vi "Get Robot Config.vi"() -> (12 "Idle Ramping Table":T1(array[cluster]), 13 "Cascade FeedForward Constants":cluster{"kA":dbl, "kS":dbl, "kG":dbl, "kV":dbl}, 14 "Manipulator Config":T2, 15 "Intake Presets":T5(array[cluster]), 16 "Scoring Overrides Ramping Table":T1(array[cluster]), 17 "Color":u32(colorbox)=8978432, 18 "Shoot Cube Config":T4, 19 "Score Ramping Table":T3(array[cluster]))   [LabVIEW 2020]
uses:
  <vilib>/Rock Robotics/Network Tables/NT Read Number.vi
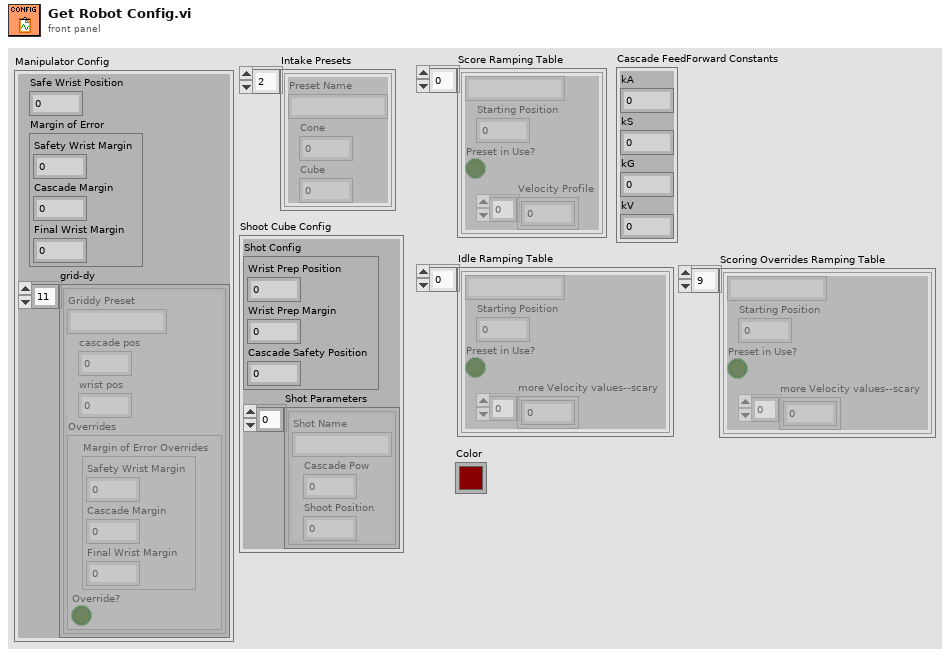
[diagram p1: front panel]
types:
  T1 = cluster{string, "Starting Position":dbl, "Preset in Use?":bool, "more Velocity values--scary":dbl[]}[]
  T2 = cluster{"Safe Wrist Position":dbl, "Margin of Error":cluster{"Safety Wrist Margin":dbl, "Cascade Margin":dbl, "Final Wrist Margin":dbl}, "grid-dy":cluster{"Griddy Preset":string, "cascade pos":dbl, "wrist pos":dbl, "Overrides":cluster{"Margin of Error Overrides":cluster{"Safety Wrist Margin":dbl, "Cascade Margin":dbl, "Final Wrist Margin":dbl}, "Override?":bool}}[]}
  T3 = cluster{string, "Starting Position":dbl, "Preset in Use?":bool, "Velocity Profile":dbl[]}[]
  T4 = cluster{"Shot Config":cluster{"Wrist Prep Position":dbl, "Wrist Prep Margin":dbl, "Cascade Safety Position":dbl}, "Shot Parameters":cluster{"Shot Name":string, "Cascade Pow":dbl, "Shoot Position":dbl}[]}
  T5 = cluster{"Preset Name":string, "Cone":dbl, "Cube":dbl}[]
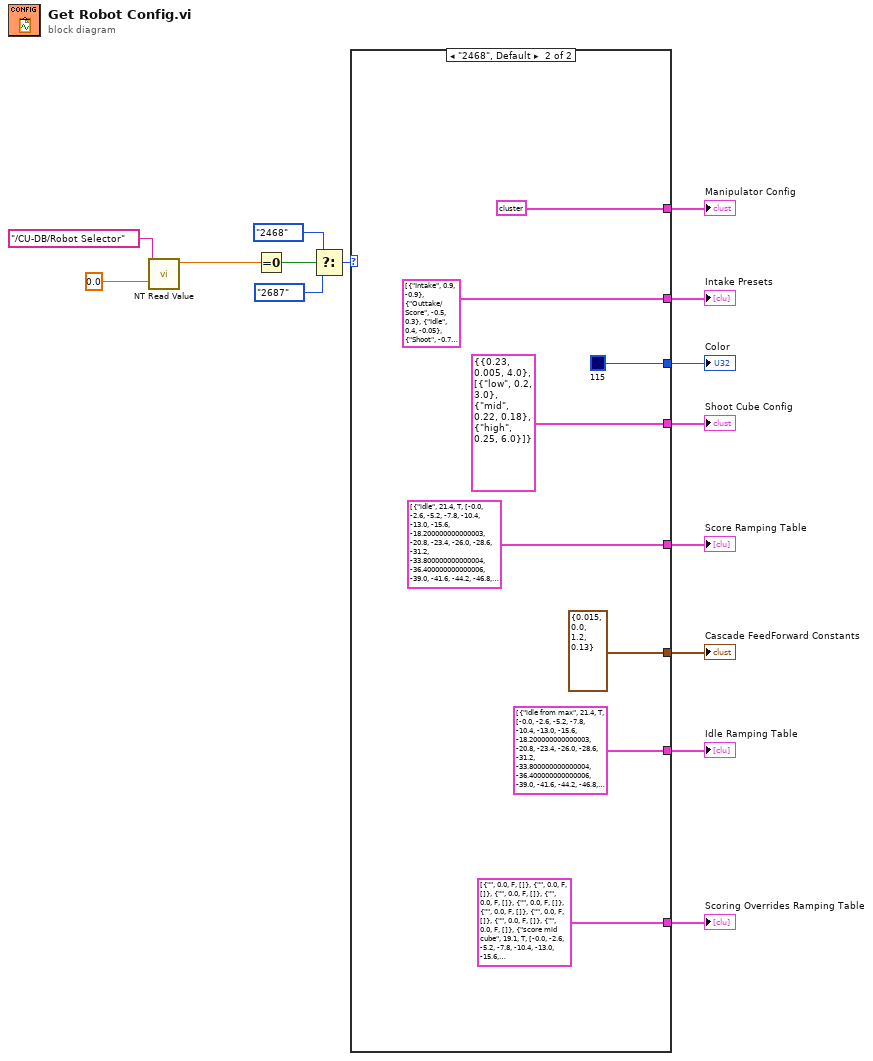
[diagram p0: block diagram]
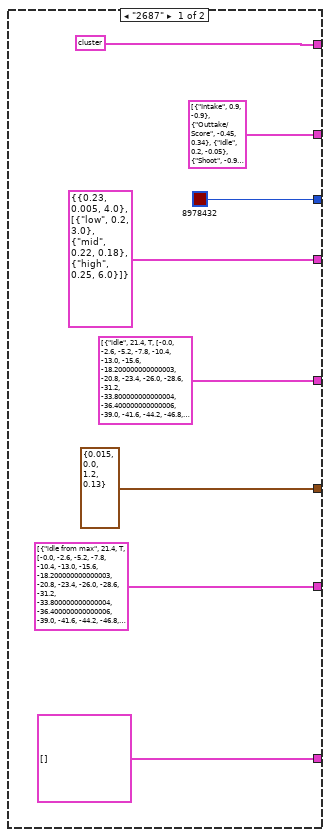
[diagram p2: hidden frame]
diagram:
  n1 = call-poly <vilib>:"NT Read Value.vi"("default value"=0.0, "name"="/CU-DB/Robot Selector") -> ("value"=w14:dbl)  [unwired: 7 in, 2 out]
  n2 = Equal To 0?(x=w14) -> (x = 0?=w13:bool)
  n3 = Select(t=enum16{"2468", "2687"}."2468", s=w13, f=enum16{"2468", "2687"}."2687") -> (s? t:f=w10:enum16{"2468", "2687"})
  n4 = case shown="\"2468\", Default" w10 {
    tunnel: [T2 {"Safe Wrist Position"=0.35, "Margin of Error"={"Safety Wrist Margin"=0.3, "Cascade Margin"=2.0, "Final Wrist Margin"=0.03}, "grid-dy"=[{"Griddy Preset"="idle", "cascade pos"=0.0, "wrist pos"=0.25, "Overrides"={"Margin of Error Overrides"={"Safety Wrist Margin"=0.3, "Cascade Margin"=2.0, "Final Wrist Margin"=0.03}, "Override?"=FALSE}}, {"Griddy Preset"="intake cone sideways", "cascade pos"=0.0, "wrist pos"=0.685, "Overrides"={"Margin of Error Overrides"={"Safety Wrist Margin"=0.3, "Cascade Margin"=2.0, "Final Wrist Margin"=0.03}, "Override?"=FALSE}}, {"Griddy Preset"="intake cone upright", "cascade pos"=6.5, "wrist pos"=0.75, "Overrides"={"Margin of Error Overrides"={"Safety Wrist Margin"=0.3, "Cascade Margin"=2.0, "Final Wrist Margin"=0.03}, "Override?"=FALSE}}, {"Griddy Preset"="intake cone feeder", "cascade pos"=0.0, "wrist pos"=0.42, "Overrides"={"Margin of Error Overrides"={"Safety Wrist Margin"=0.3, "Cascade Margin"=2.0, "Final Wrist Margin"=0.03}, "Override?"=FALSE}}, {"Griddy Preset"="intake cube feeder", "cascade pos"=0.0, "wrist pos"=0.2, "Overrides"={"Margin of Error Overrides"={"Safety Wrist Margin"=0.3, "Cascade Margin"=2.0, "Final Wrist Margin"=0.03}, "Override?"=FALSE}}, {"Griddy Preset"="intake cube", "cascade pos"=0.0, "wrist pos"=0.58, "Overrides"={"Margin of Error Overrides"={"Safety Wrist Margin"=0.3, "Cascade Margin"=2.0, "Final Wrist Margin"=0.03}, "Override?"=FALSE}}, {"Griddy Preset"="score low cone", "cascade pos"=0.0, "wrist pos"=0.5, "Overrides"={"Margin of Error Overrides"={"Safety Wrist Margin"=0.3, "Cascade Margin"=2.0, "Final Wrist Margin"=0.03}, "Override?"=FALSE}}, {"Griddy Preset"="score low cube", "cascade pos"=0.0, "wrist pos"=0.25, "Overrides"={"Margin of Error Overrides"={"Safety Wrist Margin"=0.3, "Cascade Margin"=2.0, "Final Wrist Margin"=0.03}, "Override?"=FALSE}}, {"Griddy Preset"="score mid cone", "cascade pos"=21.4, "wrist pos"=0.79, "Overrides"={"Margin of Error Overrides"={"Safety Wrist Margin"=0.3, "Cascade Margin"=13.0, "Final Wrist Margin"=0.03}, "Override?"=TRUE}}, {"Griddy Preset"="score mid cube", "cascade pos"=8.9, "wrist pos"=0.4, "Overrides"={"Margin of Error Overrides"={"Safety Wrist Margin"=0.3, "Cascade Margin"=2.0, "Final Wrist Margin"=0.03}, "Override?"=FALSE}}, {"Griddy Preset"="score high cone", "cascade pos"=21.4, "wrist pos"=0.62, "Overrides"={"Margin of Error Overrides"={"Safety Wrist Margin"=0.3, "Cascade Margin"=2.0, "Final Wrist Margin"=0.03}, "Override?"=FALSE}}, {"Griddy Preset"="score high cube", "cascade pos"=19.1, "wrist pos"=0.4, "Overrides"={"Margin of Error Overrides"={"Safety Wrist Margin"=0.3, "Cascade Margin"=2.0, "Final Wrist Margin"=0.03}, "Override?"=FALSE}}]} ("2468 Manipulator Config") T2 {"Safe Wrist Position"=0.35, "Margin of Error"={"Safety Wrist Margin"=0.3, "Cascade Margin"=2.0, "Final Wrist Margin"=0.03}, "grid-dy"=[{"Griddy Preset"="idle", "cascade pos"=0.0, "wrist pos"=0.25, "Overrides"={"Margin of Error Overrides"={"Safety Wrist Margin"=0.3, "Cascade Margin"=2.0, "Final Wrist Margin"=0.03}, "Override?"=FALSE}}, {"Griddy Preset"="intake cone sideways", "cascade pos"=0.0, "wrist pos"=0.69, "Overrides"={"Margin of Error Overrides"={"Safety Wrist Margin"=0.3, "Cascade Margin"=2.0, "Final Wrist Margin"=0.03}, "Override?"=FALSE}}, {"Griddy Preset"="intake cone upright", "cascade pos"=6.3, "wrist pos"=0.75, "Overrides"={"Margin of Error Overrides"={"Safety Wrist Margin"=0.3, "Cascade Margin"=2.0, "Final Wrist Margin"=0.03}, "Override?"=FALSE}}, {"Griddy Preset"="intake cone feeder", "cascade pos"=0.0, "wrist pos"=0.42, "Overrides"={"Margin of Error Overrides"={"Safety Wrist Margin"=0.3, "Cascade Margin"=2.0, "Final Wrist Margin"=0.03}, "Override?"=FALSE}}, {"Griddy Preset"="intake cube feeder", "cascade pos"=0.0, "wrist pos"=0.2, "Overrides"={"Margin of Error Overrides"={"Safety Wrist Margin"=0.3, "Cascade Margin"=2.0, "Final Wrist Margin"=0.03}, "Override?"=FALSE}}, {"Griddy Preset"="intake cube", "cascade pos"=0.0, "wrist pos"=0.59, "Overrides"={"Margin of Error Overrides"={"Safety Wrist Margin"=0.3, "Cascade Margin"=2.0, "Final Wrist Margin"=0.03}, "Override?"=FALSE}}, {"Griddy Preset"="score low cone", "cascade pos"=0.0, "wrist pos"=0.5, "Overrides"={"Margin of Error Overrides"={"Safety Wrist Margin"=0.3, "Cascade Margin"=2.0, "Final Wrist Margin"=0.03}, "Override?"=FALSE}}, {"Griddy Preset"="score low cube", "cascade pos"=0.0, "wrist pos"=0.25, "Overrides"={"Margin of Error Overrides"={"Safety Wrist Margin"=0.3, "Cascade Margin"=2.0, "Final Wrist Margin"=0.03}, "Override?"=FALSE}}, {"Griddy Preset"="score mid cone", "cascade pos"=21.4, "wrist pos"=0.82, "Overrides"={"Margin of Error Overrides"={"Safety Wrist Margin"=0.3, "Cascade Margin"=13.0, "Final Wrist Margin"=0.03}, "Override?"=TRUE}}, {"Griddy Preset"="score mid cube", "cascade pos"=8.9, "wrist pos"=0.38, "Overrides"={"Margin of Error Overrides"={"Safety Wrist Margin"=0.3, "Cascade Margin"=2.0, "Final Wrist Margin"=0.03}, "Override?"=FALSE}}, {"Griddy Preset"="score high cone", "cascade pos"=21.4, "wrist pos"=0.62, "Overrides"={"Margin of Error Overrides"={"Safety Wrist Margin"=0.3, "Cascade Margin"=2.0, "Final Wrist Margin"=0.03}, "Override?"=FALSE}}, {"Griddy Preset"="score high cube", "cascade pos"=19.1, "wrist pos"=0.4, "Overrides"={"Margin of Error Overrides"={"Safety Wrist Margin"=0.3, "Cascade Margin"=2.0, "Final Wrist Margin"=0.03}, "Override?"=FALSE}}]} ("2468 Manipulator Config")] -> w2
    tunnel: [T5 [{"Preset Name"="Intake", "Cone"=0.9, "Cube"=-0.9}, {"Preset Name"="Outtake/Score", "Cone"=-0.45, "Cube"=0.34}, {"Preset Name"="Idle", "Cone"=0.2, "Cube"=-0.05}, {"Preset Name"="Shoot", "Cone"=-0.9, "Cube"=0.9}] ("2687 Intake Presets") T5 [{"Preset Name"="Intake", "Cone"=0.9, "Cube"=-0.9}, {"Preset Name"="Outtake/Score", "Cone"=-0.5, "Cube"=0.3}, {"Preset Name"="Idle", "Cone"=0.4, "Cube"=-0.05}, {"Preset Name"="Shoot", "Cone"=-0.7, "Cube"=0.9}] ("2468 Intake Presets")] -> w9
    tunnel: [u32 8978432 ("Red") u32 115 ("Blue")] -> w8
    tunnel: [T4 {"Shot Config"={"Wrist Prep Position"=0.23, "Wrist Prep Margin"=0.005, "Cascade Safety Position"=4.0}, "Shot Parameters"=[{"Shot Name"="low", "Cascade Pow"=0.2, "Shoot Position"=3.0}, {"Shot Name"="mid", "Cascade Pow"=0.22, "Shoot Position"=0.18}, {"Shot Name"="high", "Cascade Pow"=0.25, "Shoot Position"=6.0}]} ("2687 Shoot Cube Config") T4 {"Shot Config"={"Wrist Prep Position"=0.23, "Wrist Prep Margin"=0.005, "Cascade Safety Position"=4.0}, "Shot Parameters"=[{"Shot Name"="low", "Cascade Pow"=0.2, "Shoot Position"=3.0}, {"Shot Name"="mid", "Cascade Pow"=0.22, "Shoot Position"=0.18}, {"Shot Name"="high", "Cascade Pow"=0.25, "Shoot Position"=6.0}]} ("2687 Shoot Cube Config")] -> w6
    tunnel: [T1 [{"idle", "Starting Position"=21.4, "Preset in Use?"=TRUE, "more Velocity values--scary"=[-0.0, -2.6, -5.2, -7.8, -10.4, -13.0, -15.6, -18.200000000000003, -20.8, -23.4, -26.0, -28.6, -31.2, -33.800000000000004, -36.400000000000006, -39.0, -41.6, -44.2, -46.8, -49.4, -52.0, -49.89880242347718, -47.29880242347717, -44.69880242347717, -42.098802423477174, -39.49880242347717, -36.89880242347717, -34.29880242347717, -31.698802423477165, -29.098802423477178, -26.498802423477176, -23.898802423477175, -21.29880242347717, -18.69880242347717, -16.098802423477167, -13.49880242347718, -10.898802423477179, -8.298802423477177, -5.698802423477169, -3.098802423477167, -0.49880242347716575]}, {"", "Starting Position"=0.0, "Preset in Use?"=FALSE, "more Velocity values--scary"=[]}, {"intake cone upright", "Starting Position"=0.0, "Preset in Use?"=TRUE, "more Velocity values--scary"=[0.0, 2.6, 5.2, 7.8, 10.4, 13.0, 15.6, 18.200000000000003, 20.8, 23.4, 26.0, 28.6, 28.26427345275879, 25.66427345275879, 23.064273452758783, 20.46427345275879, 17.864273452758788, 15.264273452758786, 12.664273452758792, 10.064273452758787, 7.4642734527587855, 4.864273452758791, 2.2642734527587898, -0.3357265472412152]}, {"", "Starting Position"=0.0, "Preset in Use?"=FALSE, "more Velocity values--scary"=[]}, {"", "Starting Position"=0.0, "Preset in Use?"=FALSE, "more Velocity values--scary"=[]}, {"", "Starting Position"=0.0, "Preset in Use?"=FALSE, "more Velocity values--scary"=[]}, {"", "Starting Position"=0.0, "Preset in Use?"=FALSE, "more Velocity values--scary"=[]}, {"", "Starting Position"=0.0, "Preset in Use?"=FALSE, "more Velocity values--scary"=[]}, {"score mid cone", "Starting Position"=0.0, "Preset in Use?"=TRUE, "more Velocity values--scary"=[0.0, 2.6, 5.2, 7.8, 10.4, 13.0, 15.6, 18.200000000000003, 20.8, 23.4, 26.0, 28.6, 31.2, 33.800000000000004, 36.400000000000006, 39.0, 41.6, 44.2, 46.8, 49.4, 49.98038995265961, 47.38038995265961, 44.780389952659604, 42.1803899526596, 39.58038995265961, 36.98038995265961, 34.380389952659606, 31.780389952659604, 29.1803899526596, 26.580389952659612, 23.98038995265961, 21.38038995265961, 18.780389952659604, 16.180389952659603, 13.580389952659601, 10.980389952659614, 8.380389952659613, 5.780389952659611, 3.1803899526596027, 0.5803899526596012]}, {"score mid cube", "Starting Position"=0.0, "Preset in Use?"=TRUE, "more Velocity values--scary"=[0.0, 2.6, 5.2, 7.8, 10.4, 13.0, 15.6, 18.200000000000003, 20.8, 23.4, 26.0, 28.6, 31.2, 32.683082771301265, 30.083082771301267, 27.48308277130127, 24.883082771301268, 22.283082771301267, 19.683082771301272, 17.083082771301267, 14.483082771301266, 11.883082771301272, 9.28308277130127, 6.683082771301265, 4.083082771301271, 1.4830827713012695, -1.116917228698732]}, {"score high cone", "Starting Position"=0.0, "Preset in Use?"=TRUE, "more Velocity values--scary"=[0.0, 1.6, 3.2, 4.8, 6.4, 8.0, 9.6, 11.200000000000001, 12.8, 14.399999999999999, 16.0, 17.6, 19.2, 20.8, 22.400000000000002, 24.0, 25.6, 27.200000000000003, 28.799999999999997, 30.4, 32.0, 33.6, 35.2, 36.800000000000004, 38.4, 40.0, 41.15264739990234, 39.55264739990234, 37.95264739990234, 36.352647399902345, 34.752647399902344, 33.15264739990234, 31.55264739990234, 29.95264739990234, 28.352647399902338, 26.752647399902347, 25.152647399902346, 23.552647399902344, 21.952647399902343, 20.35264739990234, 18.75264739990234, 17.15264739990235, 15.552647399902348, 13.952647399902347, 12.352647399902345, 10.752647399902344, 9.152647399902342, 7.552647399902348, 5.952647399902347, 4.352647399902345, 2.7526473999023438, 1.1526473999023423, -0.4473526000976591]}, {"score high cube", "Starting Position"=0.0, "Preset in Use?"=TRUE, "more Velocity values--scary"=[0.0, 2.6, 5.2, 7.8, 10.4, 13.0, 15.6, 18.200000000000003, 20.8, 23.4, 26.0, 28.6, 31.2, 33.800000000000004, 36.400000000000006, 39.0, 41.6, 44.2, 46.8, 49.4, 47.39819097518921, 44.798190975189215, 42.198190975189206, 39.598190975189205, 36.99819097518921, 34.39819097518921, 31.798190975189208, 29.198190975189206, 26.5981909751892, 23.998190975189214, 21.398190975189213, 18.79819097518921, 16.198190975189206, 13.598190975189205, 10.998190975189203, 8.398190975189216, 5.798190975189215, 3.1981909751892132, 0.5981909751892047]}] ("2687 Score Ramping Table") T1 [{"idle", "Starting Position"=21.4, "Preset in Use?"=TRUE, "more Velocity values--scary"=[-0.0, -2.6, -5.2, -7.8, -10.4, -13.0, -15.6, -18.200000000000003, -20.8, -23.4, -26.0, -28.6, -31.2, -33.800000000000004, -36.400000000000006, -39.0, -41.6, -44.2, -46.8, -49.4, -52.0, -49.89880242347718, -47.29880242347717, -44.69880242347717, -42.098802423477174, -39.49880242347717, -36.89880242347717, -34.29880242347717, -31.698802423477165, -29.098802423477178, -26.498802423477176, -23.898802423477175, -21.29880242347717, -18.69880242347717, -16.098802423477167, -13.49880242347718, -10.898802423477179, -8.298802423477177, -5.698802423477169, -3.098802423477167, -0.49880242347716575]}, {"", "Starting Position"=0.0, "Preset in Use?"=FALSE, "more Velocity values--scary"=[]}, {"intake cone upright", "Starting Position"=0.0, "Preset in Use?"=TRUE, "more Velocity values--scary"=[0.0, 1.26, 2.52, 3.78, 5.04, 6.300000000000001, 7.56, 8.82, 10.08, 11.34, 12.600000000000001, 13.86, 15.12, 16.38, 17.64, 18.9, 19.68469825029373, 18.42469825029373, 17.164698250293732, 15.90469825029373, 14.64469825029373, 13.384698250293733, 12.124698250293733, 10.864698250293731, 9.604698250293733, 8.344698250293732, 7.08469825029373, 5.824698250293729, 4.564698250293729, 3.3046982502937325, 2.0446982502937345, 0.784698250293733, -0.4753017497062686]}, {"", "Starting Position"=0.0, "Preset in Use?"=FALSE, "more Velocity values--scary"=[]}, {"", "Starting Position"=0.0, "Preset in Use?"=FALSE, "more Velocity values--scary"=[]}, {"", "Starting Position"=0.0, "Preset in Use?"=FALSE, "more Velocity values--scary"=[]}, {"", "Starting Position"=0.0, "Preset in Use?"=FALSE, "more Velocity values--scary"=[]}, {"", "Starting Position"=0.0, "Preset in Use?"=FALSE, "more Velocity values--scary"=[]}, {"score mid cone", "Starting Position"=0.0, "Preset in Use?"=TRUE, "more Velocity values--scary"=[0.0, 1.26, 2.52, 3.78, 5.04, 6.300000000000001, 7.56, 8.82, 10.08, 11.34, 12.600000000000001, 13.86, 15.12, 16.38, 17.64, 18.9, 20.16, 21.42, 22.68, 23.94, 25.200000000000003, 26.459999999999997, 27.72, 28.98, 30.24, 31.5, 32.76, 34.02, 35.28, 36.54, 35.63568778038025, 34.37568778038025, 33.11568778038025, 31.855687780380247, 30.595687780380246, 29.33568778038025, 28.07568778038025, 26.81568778038025, 25.555687780380246, 24.29568778038025, 23.035687780380247, 21.775687780380252, 20.51568778038025, 19.25568778038025, 17.995687780380248, 16.735687780380246, 15.475687780380248, 14.215687780380254, 12.955687780380252, 11.69568778038025, 10.435687780380249, 9.175687780380247, 7.915687780380246, 6.655687780380244, 5.395687780380243, 4.135687780380245, 2.8756877803802396, 1.6156877803802558, 0.35568778038025073]}, {"score mid cube", "Starting Position"=0.0, "Preset in Use?"=TRUE, "more Velocity values--scary"=[0.0, 1.26, 2.52, 3.78, 5.04, 6.300000000000001, 7.56, 8.82, 10.08, 11.34, 12.600000000000001, 13.86, 15.12, 16.38, 17.64, 18.9, 20.16, 21.42, 22.68, 23.418210504055022, 22.15821050405502, 20.898210504055022, 19.638210504055024, 18.378210504055023, 17.118210504055025, 15.858210504055023, 14.598210504055022, 13.33821050405502, 12.07821050405502, 10.818210504055026, 9.558210504055024, 8.298210504055023, 7.038210504055023, 5.778210504055021, 4.51821050405502, 3.2582105040550253, 1.9982105040550238, 0.7382105040550222, -0.5217894959449758]}, {"score high cone", "Starting Position"=0.0, "Preset in Use?"=TRUE, "more Velocity values--scary"=[0.0, 1.26, 2.52, 3.78, 5.04, 6.300000000000001, 7.56, 8.82, 10.08, 11.34, 12.600000000000001, 13.86, 15.12, 16.38, 17.64, 18.9, 20.16, 21.42, 22.68, 23.94, 25.200000000000003, 26.459999999999997, 27.72, 28.98, 30.24, 31.5, 32.76, 34.02, 35.28, 36.54, 35.63568778038025, 34.37568778038025, 33.11568778038025, 31.855687780380247, 30.595687780380246, 29.33568778038025, 28.07568778038025, 26.81568778038025, 25.555687780380246, 24.29568778038025, 23.035687780380247, 21.775687780380252, 20.51568778038025, 19.25568778038025, 17.995687780380248, 16.735687780380246, 15.475687780380248, 14.215687780380254, 12.955687780380252, 11.69568778038025, 10.435687780380249, 9.175687780380247, 7.915687780380246, 6.655687780380244, 5.395687780380243, 4.135687780380245, 2.8756877803802396, 1.6156877803802558, 0.35568778038025073]}, {"score high cube", "Starting Position"=0.0, "Preset in Use?"=TRUE, "more Velocity values--scary"=[0.0, 1.26, 2.52, 3.78, 5.04, 6.300000000000001, 7.56, 8.82, 10.08, 11.34, 12.600000000000001, 13.86, 15.12, 16.38, 17.64, 18.9, 20.16, 21.42, 22.68, 23.94, 25.200000000000003, 26.459999999999997, 27.72, 28.98, 30.24, 31.5, 32.76, 34.02, 34.09722873687744, 32.83722873687744, 31.577228736877444, 30.317228736877443, 29.05722873687744, 27.79722873687744, 26.537228736877438, 25.277228736877444, 24.017228736877442, 22.757228736877444, 21.49722873687744, 20.23722873687744, 18.97722873687744, 17.717228736877445, 16.457228736877443, 15.197228736877442, 13.93722873687744, 12.677228736877439, 11.41722873687744, 10.157228736877446, 8.897228736877445, 7.637228736877443, 6.377228736877441, 5.11722873687744, 3.8572287368774383, 2.5972287368774403, 1.3372287368774352, 0.07722873687743714]}] ("2687 Score Ramping Table")] -> w5
    tunnel: [cluster{"kA":dbl, "kS":dbl, "kG":dbl, "kV":dbl} {"kA"=0.015, "kS"=0.0, "kG"=1.2, "kV"=0.13} ("2687 FeedForward Constants") cluster{"kA":dbl, "kS":dbl, "kG":dbl, "kV":dbl} {"kA"=0.015, "kS"=0.0, "kG"=1.2, "kV"=0.13} ("2687 FeedForward Constants")] -> w4
    tunnel: [T1 [{"idle from max", "Starting Position"=21.4, "Preset in Use?"=TRUE, "more Velocity values--scary"=[-0.0, -2.6, -5.2, -7.8, -10.4, -13.0, -15.6, -18.200000000000003, -20.8, -23.4, -26.0, -28.6, -31.2, -33.800000000000004, -36.400000000000006, -39.0, -41.6, -44.2, -46.8, -49.4, -52.0, -50.889337444305426, -48.28933744430542, -45.689337444305416, -43.08933744430542, -40.48933744430542, -37.88933744430542, -35.28933744430542, -32.68933744430541, -30.089337444305425, -27.489337444305423, -24.889337444305422, -22.289337444305417, -19.689337444305416, -17.089337444305414, -14.489337444305427, -11.889337444305426, -9.289337444305424, -6.689337444305416, -4.089337444305414, -1.4893374443054128, 1.1106625556945744]}, {"idle from high cube", "Starting Position"=19.4, "Preset in Use?"=TRUE, "more Velocity values--scary"=[-0.0, -2.6, -5.2, -7.8, -10.4, -13.0, -15.6, -18.200000000000003, -20.8, -23.4, -26.0, -28.6, -31.2, -33.800000000000004, -36.400000000000006, -39.0, -41.6, -44.2, -46.8, -49.4, -47.39819097518921, -44.798190975189215, -42.198190975189206, -39.598190975189205, -36.99819097518921, -34.39819097518921, -31.798190975189208, -29.198190975189206, -26.5981909751892, -23.998190975189214, -21.398190975189213, -18.79819097518921, -16.198190975189206, -13.598190975189205, -10.998190975189203, -8.398190975189216, -5.798190975189215, -3.1981909751892132, -0.5981909751892047]}, {"idle mid cube", "Starting Position"=8.7, "Preset in Use?"=TRUE, "more Velocity values--scary"=[-0.0, -2.6, -5.2, -7.8, -10.4, -13.0, -15.6, -18.200000000000003, -20.8, -23.4, -26.0, -28.6, -31.2, -32.683082771301265, -30.083082771301267, -27.48308277130127, -24.883082771301268, -22.283082771301267, -19.683082771301272, -17.083082771301267, -14.483082771301266, -11.883082771301272, -9.28308277130127, -6.683082771301265, -4.083082771301271, -1.4830827713012695, 1.116917228698732]}, {"idle upright cone", "Starting Position"=6.8, "Preset in Use?"=TRUE, "more Velocity values--scary"=[-0.0, -2.6, -5.2, -7.8, -10.4, -13.0, -15.6, -18.200000000000003, -20.8, -23.4, -26.0, -28.6, -28.26427345275879, -25.66427345275879, -23.064273452758783, -20.46427345275879, -17.864273452758788, -15.264273452758786, -12.664273452758792, -10.064273452758787, -7.4642734527587855, -4.864273452758791, -2.2642734527587898, 0.3357265472412152]}] ("2687 Idle Ramping Table") T1 [{"idle from max", "Starting Position"=21.4, "Preset in Use?"=TRUE, "more Velocity values--scary"=[-0.0, -2.6, -5.2, -7.8, -10.4, -13.0, -15.6, -18.200000000000003, -20.8, -23.4, -26.0, -28.6, -31.2, -33.800000000000004, -36.400000000000006, -39.0, -41.6, -44.2, -46.8, -49.4, -52.0, -50.889337444305426, -48.28933744430542, -45.689337444305416, -43.08933744430542, -40.48933744430542, -37.88933744430542, -35.28933744430542, -32.68933744430541, -30.089337444305425, -27.489337444305423, -24.889337444305422, -22.289337444305417, -19.689337444305416, -17.089337444305414, -14.489337444305427, -11.889337444305426, -9.289337444305424, -6.689337444305416, -4.089337444305414, -1.4893374443054128, 1.1106625556945744]}, {"idle from high cube", "Starting Position"=19.1, "Preset in Use?"=TRUE, "more Velocity values--scary"=[-0.0, -2.6, -5.2, -7.8, -10.4, -13.0, -15.6, -18.200000000000003, -20.8, -23.4, -26.0, -28.6, -31.2, -33.800000000000004, -36.400000000000006, -39.0, -41.6, -44.2, -46.8, -49.4, -47.659419655799866, -45.05941965579987, -42.45941965579986, -39.85941965579986, -37.25941965579987, -34.659419655799866, -32.059419655799864, -29.459419655799863, -26.859419655799858, -24.25941965579987, -21.65941965579987, -19.059419655799868, -16.459419655799863, -13.859419655799861, -11.25941965579986, -8.659419655799873, -6.059419655799871, -3.45941965579987, -0.8594196557998615]}, {"idle mid cube", "Starting Position"=8.9, "Preset in Use?"=TRUE, "more Velocity values--scary"=[-0.0, -2.6, -5.2, -7.8, -10.4, -13.0, -15.6, -18.200000000000003, -20.8, -23.4, -26.0, -28.6, -31.2, -33.800000000000004, -31.629401898384092, -29.029401898384094, -26.429401898384093, -23.82940189838409, -21.229401898384097, -18.629401898384096, -16.02940189838409, -13.429401898384096, -10.829401898384095, -8.22940189838409, -5.629401898384096, -3.0294018983840942, -0.4294018983840928]}, {"idle upright cone", "Starting Position"=6.3, "Preset in Use?"=TRUE, "more Velocity values--scary"=[-0.0, -2.6, -5.2, -7.8, -10.4, -13.0, -15.6, -18.200000000000003, -20.8, -23.4, -26.0, -28.6, -26.036352264881135, -23.436352264881133, -20.83635226488113, -18.236352264881134, -15.636352264881133, -13.036352264881131, -10.436352264881137, -7.836352264881132, -5.2363522648811305, -2.636352264881136, -0.036352264881134744]}] ("2687 Idle Ramping Table")] -> w3
    tunnel: [T1 [] ("Scoring Overrides Ramping Table") T1 [{"", "Starting Position"=0.0, "Preset in Use?"=FALSE, "more Velocity values--scary"=[]}, {"", "Starting Position"=0.0, "Preset in Use?"=FALSE, "more Velocity values--scary"=[]}, {"", "Starting Position"=0.0, "Preset in Use?"=FALSE, "more Velocity values--scary"=[]}, {"", "Starting Position"=0.0, "Preset in Use?"=FALSE, "more Velocity values--scary"=[]}, {"", "Starting Position"=0.0, "Preset in Use?"=FALSE, "more Velocity values--scary"=[]}, {"", "Starting Position"=0.0, "Preset in Use?"=FALSE, "more Velocity values--scary"=[]}, {"", "Starting Position"=0.0, "Preset in Use?"=FALSE, "more Velocity values--scary"=[]}, {"", "Starting Position"=0.0, "Preset in Use?"=FALSE, "more Velocity values--scary"=[]}, {"", "Starting Position"=0.0, "Preset in Use?"=FALSE, "more Velocity values--scary"=[]}, {"score mid cube", "Starting Position"=19.1, "Preset in Use?"=TRUE, "more Velocity values--scary"=[-0.0, -2.6, -5.2, -7.8, -10.4, -13.0, -15.6, -18.200000000000003, -20.8, -23.4, -26.0, -28.6, -31.2, -33.800000000000004, -36.400000000000006, -33.828569412231445, -31.228569412231444, -28.628569412231442, -26.028569412231448, -23.428569412231447, -20.82856941223144, -18.228569412231447, -15.628569412231446, -13.028569412231441, -10.428569412231447, -7.828569412231445, -5.228569412231444, -2.6285694122314425, -0.02856941223144105]}, {"", "Starting Position"=0.0, "Preset in Use?"=FALSE, "more Velocity values--scary"=[]}, {"score high cube", "Starting Position"=8.9, "Preset in Use?"=TRUE, "more Velocity values--scary"=[0.0, 1.6, 3.2, 4.8, 6.4, 8.0, 9.6, 11.200000000000001, 12.8, 14.399999999999999, 16.0, 17.6, 19.2, 20.8, 22.400000000000002, 24.0, 25.6, 27.200000000000003, 28.331428718566897, 26.731428718566896, 25.131428718566895, 23.531428718566897, 21.931428718566895, 20.331428718566894, 18.731428718566896, 17.131428718566895, 15.531428718566893, 13.931428718566892, 12.33142871856689, 10.731428718566896, 9.131428718566895, 7.531428718566893, 5.931428718566892, 4.33142871856689, 2.731428718566889, 1.131428718566898, -0.46857128143310334]}] ("2468 Scoring Overrides Ramping Table")] -> w1
    frame "2687" {
    }
    frame "2468", Default {
    }
  }
  "Intake Presets" <- w9
  "Color" <- w8
  "Shoot Cube Config" <- w6
  "Score Ramping Table" <- w5
  "Cascade FeedForward Constants" <- w4
  "Idle Ramping Table" <- w3
  "Manipulator Config" <- w2
  "Scoring Overrides Ramping Table" <- w1
